vi "core_RunningAllanMain.vi"(8 "error in (no error)":errorcluster, 9 "input data point":dbl, 11 "RunningAllanCarry in":T1) -> (0 "error out":errorcluster, 1 "allanDevs":dbl[](array[numeric]), 2 "lengths":i32[](array[numeric]), 3 "RunningAllanCarry out":T1)   [LabVIEW 2015]
uses:
  core_RunningAllanCarry.vi
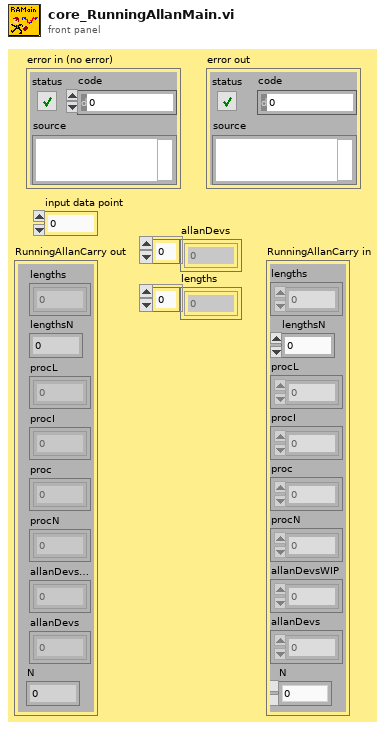
[diagram p1: front panel]
types:
  T1 = typedef "core_RunningAllanCarry.vi" = cluster{"lengths":i32[], "lengthsN":i32, "procL":i32[], "procI":i32[], "proc":dbl[], "procN":i32[], "allanDevsWIP":dbl[], "allanDevs":dbl[], "N":i32}
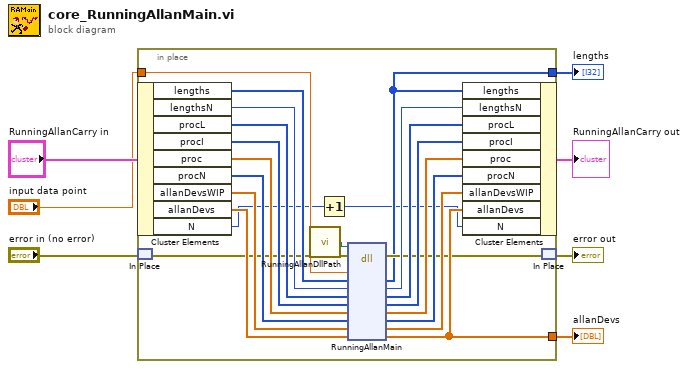
[diagram p0: block diagram]
diagram:
  n1 = in-place {
    in-place-border: [w14] -> w5
    in-place-border: "input data point" -> [w13]
    in-place-border: [w10] -> w1
    n2 = in-place-cluster #1("RunningAllanCarry in") -> ("lengths"=w28:i32[], "lengthsN"=w27:i32, "procL"=w26:i32[], "procI"=w25:i32[], "proc"=w24:dbl[], "procN"=w23:i32[], "allanDevsWIP"=w22:dbl[], "allanDevs"=w21:dbl[], "N"=w9:i32)
    n3 = in-place-match #2("error in (no error)") -> (w12:errorcluster)
    n4 = call "RunningAllanDllPath.vi"() -> ("dll path"=w29:path)
    n5 = Increment(x=w9) -> (x+1=w8:i32)
    n6 = dll-call lib="C:/Users/srmgroup/CEAS v1/utils/average_tools/cores/RunningAllanCpp/RunningAllan.dll" fn="RunningAllanMain"(path in=w29, error in=w12, "input"=w13, "lengths"=w28, "lengthsN"=w27, "procL"=w26, "procI"=w25, "proc"=w24, "procN"=w23, "allanDevsWIP"=w22, "allanDevs"=w21) -> (error out=w11:errorcluster, "lengths"=w10:i32[], "lengthsN"=w20:i32, "procL"=w19:i32[], "procI"=w18:i32[], "proc"=w17:dbl[], "procN"=w16:i32[], "allanDevsWIP"=w15:dbl[], "allanDevs"=w14:dbl[])  [unwired: 3 in, 1 out]
    n7 = in-place-cluster #1("lengths"=w10, "lengthsN"=w20, "procL"=w19, "procI"=w18, "proc"=w17, "procN"=w16, "allanDevsWIP"=w15, "allanDevs"=w14, "N"=w8) -> (→"RunningAllanCarry out":T1)
    n8 = in-place-match #2(w11) -> (→"error out":errorcluster)
  }
  "allanDevs" <- w5
  "lengths" <- w1
